vi "单轴运动.vi"() -> ()   [LabVIEW 2012]
panel:
  in  "停止速度":dbl=100.0
  out "运行曲线图 2":cluster{dbl[], i32[]}[](graph)
  out "运行时间":dbl
  out "当前状态":string
  out "当前速度":dbl
  out "当前位置":i32
  out "运行曲线图":cluster{dbl[], dbl[]}[](graph)
  in  "在线变位":bool
  in  "变位的位置值":i32=21000
  in  "平滑时间ms":dbl
  in  "减速时间s":dbl=0.5
  in  "加速时间s":dbl=0.5
  in  "运行速度":dbl=100000.0
  in  "起始速度":dbl=500.0
  in  "变速的速度值":dbl=1500.0
  in  "运动模式":enum32{"相对", "绝对"}(radio)
  in  "运动距离":i32=300000
  in  "运动方式":enum32{"点位", "连续"}(radio)
  in  "运动方向":enum32{"正向", "反向"}(radio)
  in  "在线变速":bool
  in  "退出":bool
  in  "紧急停止":bool
  in  "减速停止":bool
  in  "运行":bool
  in  "轴号选择":T1(ring)
  in  "脉冲清零":bool
  in  "卡号选择":u16(ring) items=["0"]
  out "init":bool
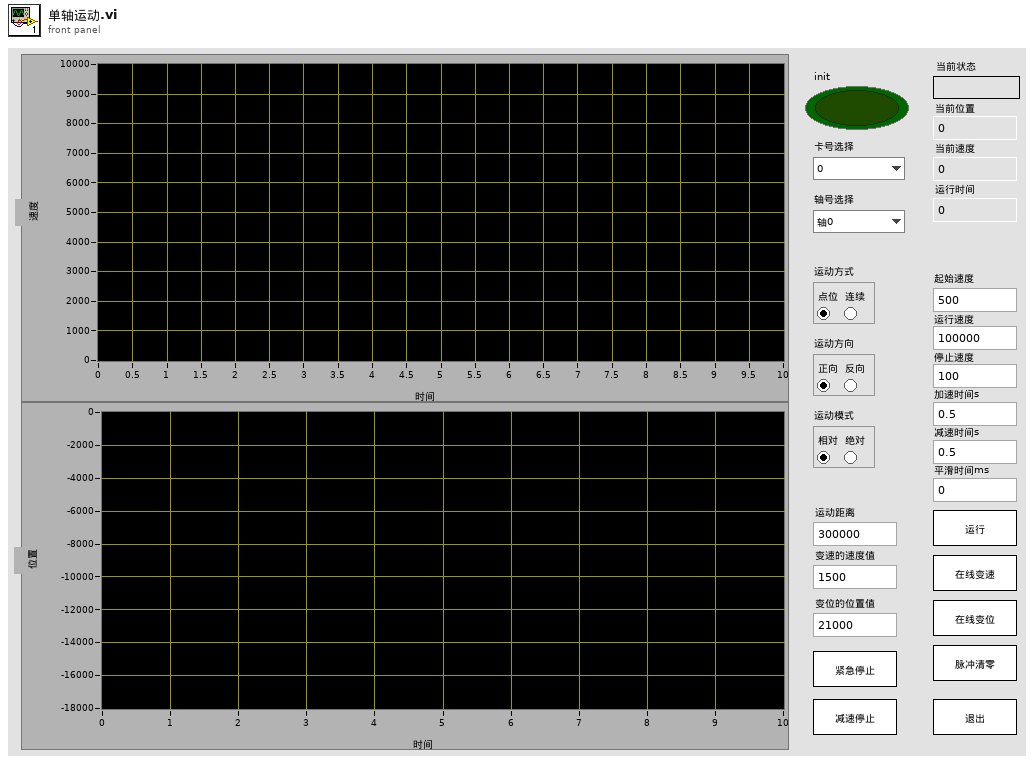
[diagram p1: front panel]
types:
  T1 = enum16{"轴0", "轴1", "轴2", "轴3", "轴4", "轴5", "轴6", "轴7"}
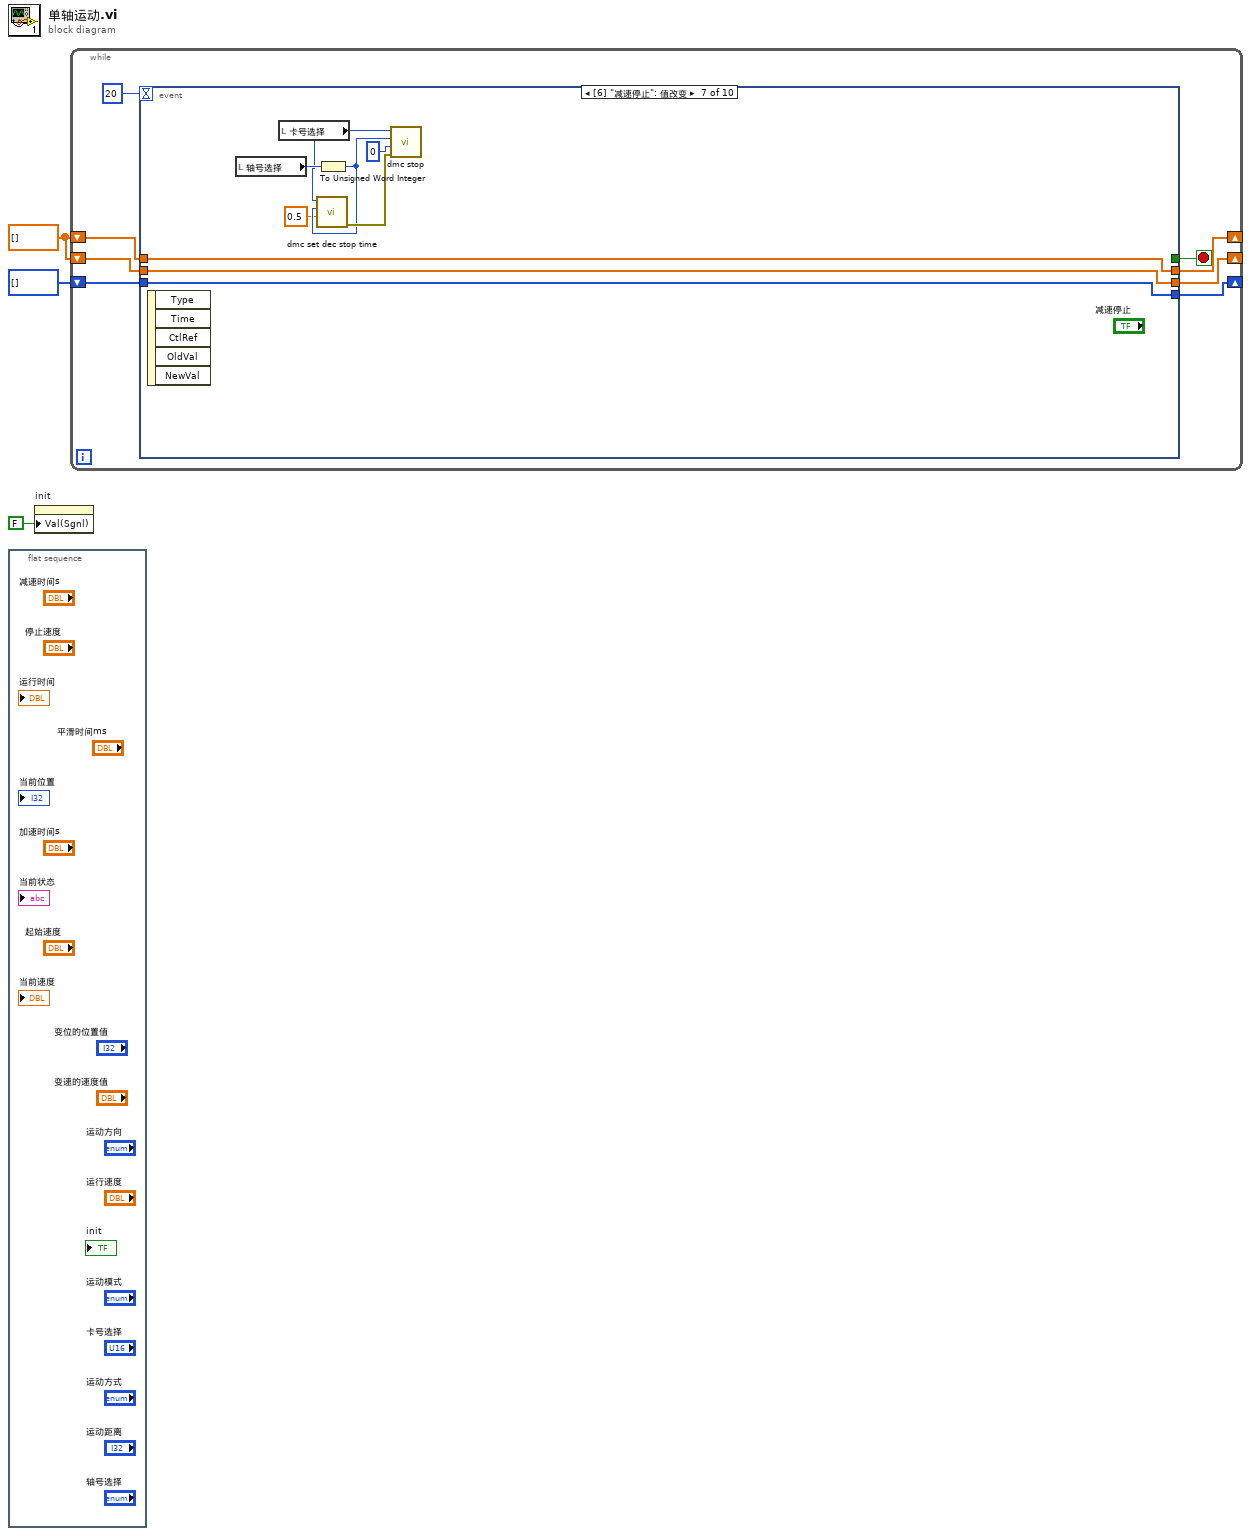
[diagram p0: block diagram]
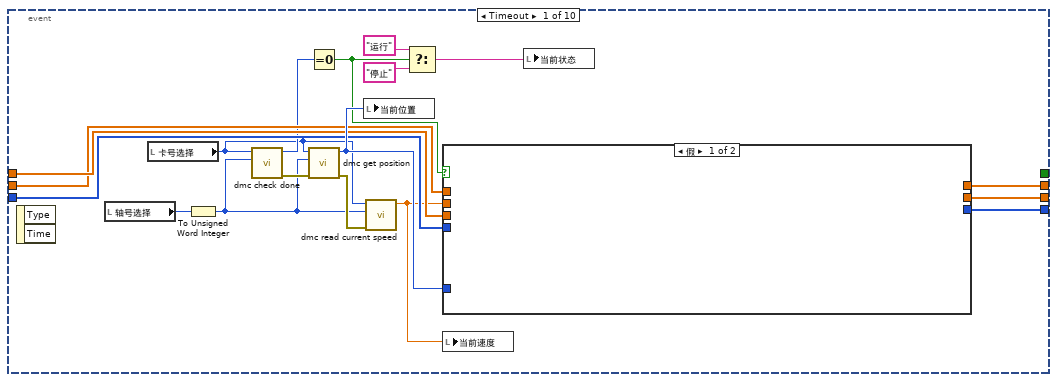
[diagram p2: hidden frame]
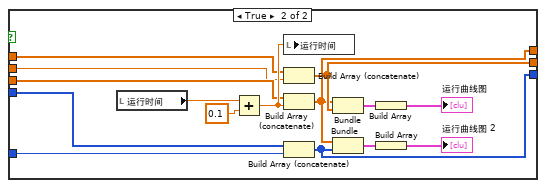
[diagram p3: hidden frame]
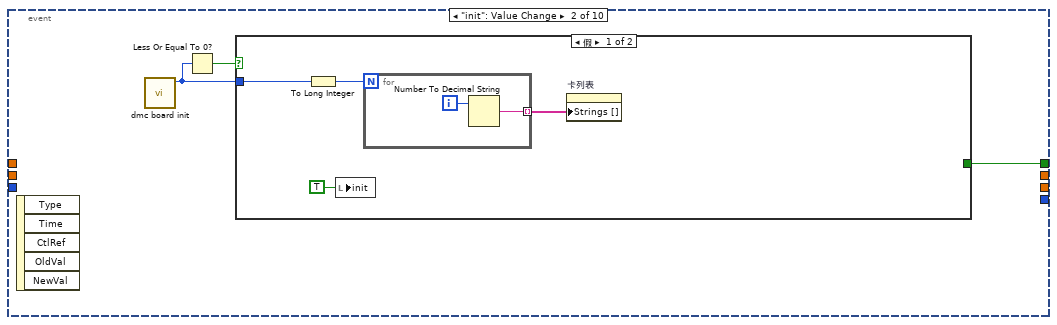
[diagram p4: hidden frame]
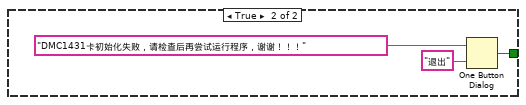
[diagram p5: hidden frame]
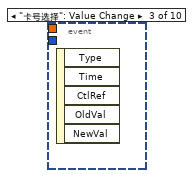
[diagram p6: hidden frame]
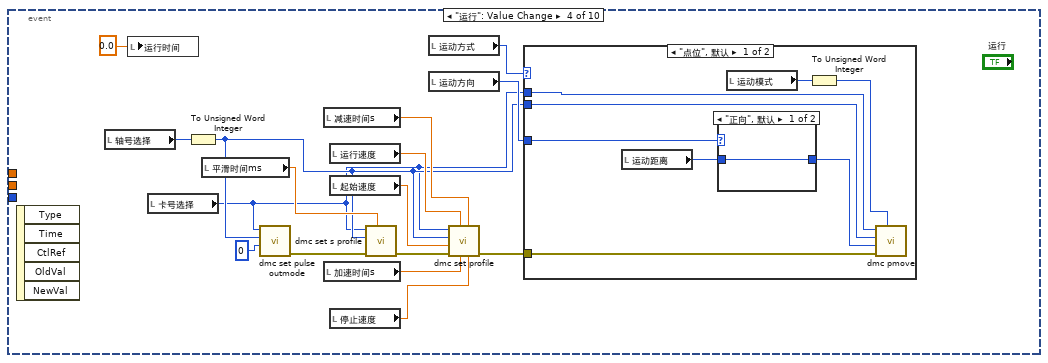
[diagram p7: hidden frame]
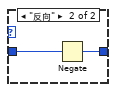
[diagram p8: hidden frame]
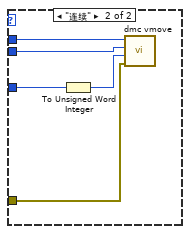
[diagram p9: hidden frame]
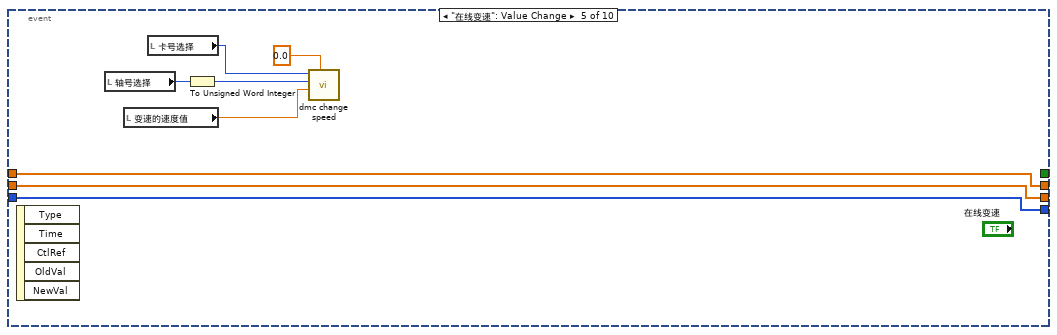
[diagram p10: hidden frame]
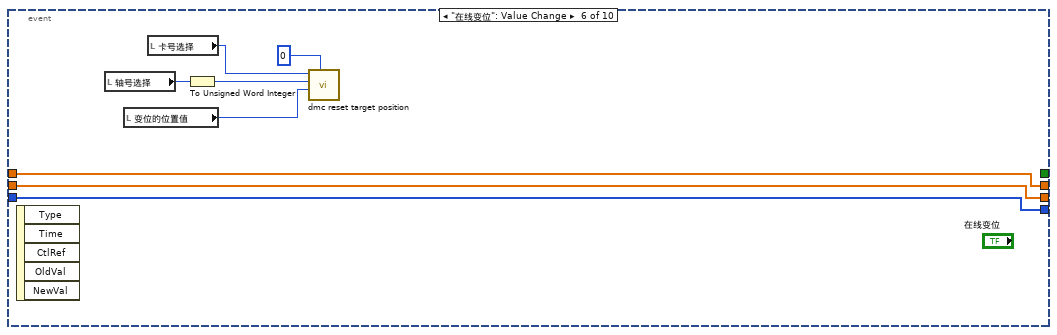
[diagram p11: hidden frame]
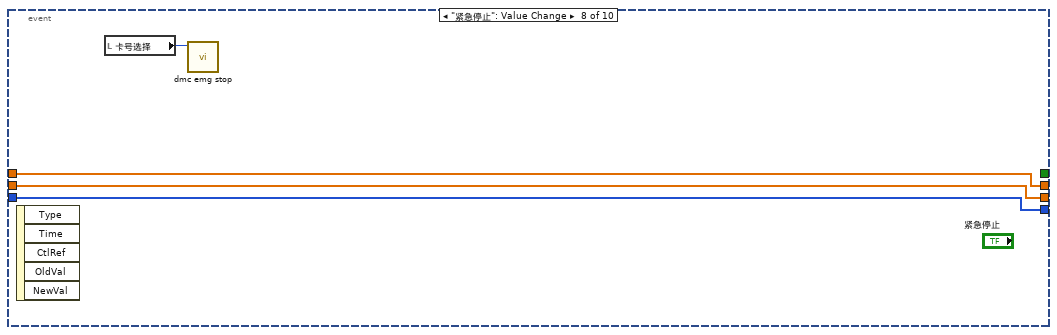
[diagram p12: hidden frame]
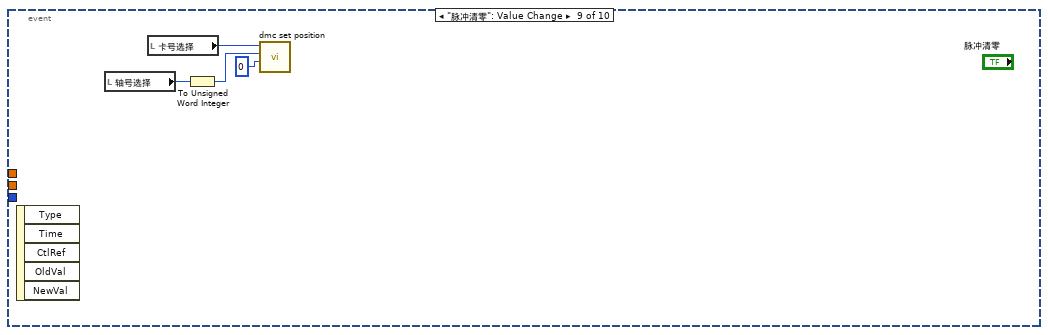
[diagram p13: hidden frame]
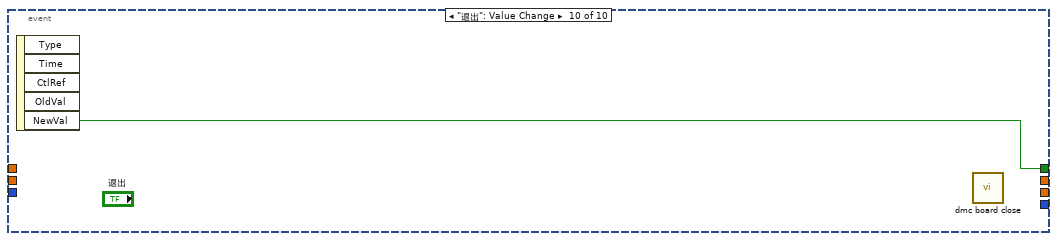
[diagram p14: hidden frame]
diagram:
  w1 = dbl[] []
  n1 = flat-sequence {
    frame #0 {
    }
  }
  n2 = property on="init" class="Bool (严格)"("Val(Sgnl)"=FALSE ("值(信号)")) -> ()  [unwired: 2 in, 2 out]
  n3 = while {
    shift-right: [w9] -> _
    shift-left: w1 -> [w8]
    shift-right: [w7] -> _
    shift-left: i32[] [] -> [w6]
    shift-right: [w4] -> _
    shift-left: w1 -> [w5]
    stop <- w11 stop-if-true
    n4 = event shown="[6] \"减速停止\": 值改变" {
      selector: _ -> [_ _ _ _ _ _ _ _ _ _]
      dyn-events: _ -> [_ _ _ _ _ _ _ _ _ _]
      timeout: 20 -> [_ _ _ _ _ _ _ _ _ _]
      tunnel: [_ w46 _ _ _ _ _ _ _ w122] -> w11
      tunnel: [w24 _ _ _ w95 w103 w112 w117 _ _] -> w9
      tunnel: w8 -> [w23 _ _ _ w95 w103 w112 w117 _ _]
      tunnel: [w22 _ _ _ w94 w102 w111 w116 _ _] -> w7
      tunnel: w6 -> [w21 _ _ _ w94 w102 w111 w116 _ _]
      tunnel: w5 -> [w20 _ _ _ w93 w101 w110 w115 _ _]
      tunnel: [w19 _ _ _ w93 w101 w110 w115 _ _] -> w4
      event Timeout {
        n5 = event-data() -> ()  [unwired: 1 in, 2 out]
        n6 = local read "轴号选择"() -> (w29:T1)
        n7 = local read "卡号选择"() -> (w13:u16)
        n8 = To Unsigned Word Integer(number=w29) -> (unsigned 16bit integer=w12:u16)
        n9 = call "dmc check done.vi"("axis"=w12, "CardNo"=w13) -> ("error out"=w15:errorcluster, "function return"=w16:i16)  [unwired: 8 in]
        n10 = Equal To 0?(x=w16) -> (x = 0?=w17:bool)
        n11 = call "dmc get position.vi"("error in (no error)"=w15, "axis"=w12, "CardNo"=w13) -> ("error out"=w14:errorcluster, "function return"=w25:i32)  [unwired: 7 in]
        n12 = local write "当前位置"(w25) -> ()
        n13 = call "dmc read current speed.vi"("error in (no error)"=w14, "axis"=w12, "CardNo"=w13) -> ("function return"=w18:dbl)  [unwired: 7 in, 1 out]
        n14 = Select(t="运行" ("当前状态"), s=w17, f="停止" ("当前状态")) -> (s? t:f=w28:string)
        n15 = case shown="假" w17 {
          tunnel: w25 -> [_ w40]
          tunnel: [_ w34] -> w24
          tunnel: w23 -> [_ w41]
          tunnel: [_ w38] -> w22
          tunnel: w21 -> [_ w39]
          tunnel: w20 -> [_ w37]
          tunnel: [_ w35] -> w19
          tunnel: w18 -> [_ w36]
          frame False {
          }
          frame True {
            n16 = local read "运行时间"() -> (w44:dbl)
            n17 = Add(x=w44, y=0.1) -> (x+y=w42:dbl)
            n18 = local write "运行时间"(w42) -> ()
            n19 = Build Array (concatenate)(w37, w36) -> (w35:dbl[])
            n20 = Build Array (concatenate)(w41, w42) -> (w34:dbl[])
            n21 = Build Array (concatenate)(w39, w40) -> (w38:i32[])
            n22 = Bundle(w34, w35) -> (w33:cluster{dbl[], dbl[]})  [unwired: 1 in]
            n23 = Bundle(w34, w38) -> (w30:cluster{dbl[], i32[]})  [unwired: 1 in]
            n24 = Build Array(w33) -> (→"运行曲线图":cluster{dbl[], dbl[]}[])
            n25 = Build Array(w30) -> (→"运行曲线图 2":cluster{dbl[], i32[]}[])
          }
        }
        n26 = local write "当前速度"(w18) -> ()
        n27 = local write "当前状态"(w28) -> ()
      }
      event "init": Value Change {
        n28 = event-data() -> ()  [unwired: 1 in, 5 out]
        n29 = call "dmc board init.vi"() -> ("function return"=w45:i16)  [unwired: 10 in, 1 out]
        n30 = Less Or Equal To 0?(x=w45) -> (x <= 0?=w47:bool)
        n31 = case shown="假" w47 {
          tunnel: [_ w54] -> w46
          tunnel: w45 -> [w51 _]
          frame False {
            n32 = To Long Integer(number=w51) -> (32bit integer=w50:i32)
            n33 = local write "init"(TRUE ("init")) -> ()
            n34 = for {
              N: w50 -> [_]
              tunnel: [w52] -> w49 mode=indexing
              i -> [w53]
              n35 = Number To Decimal String(number=w53) -> (decimal integer string=w52:string)  [unwired: 1 in]
            }
            n36 = property on="卡列表" class="Ring (严格)"("Strings []"=w49) -> ()  [unwired: 2 in, 2 out]
          }
          frame True {
            n37 = One Button Dialog(message="DMC1431卡初始化失败，请检查后再尝试运行程序，谢谢！！！" ("消息"), button name ("OK")="退出" ("按钮名称（“确定”）")) -> (true=w54:bool)
          }
        }
      }
      event "卡号选择": Value Change {
        n38 = event-data() -> ()  [unwired: 1 in, 5 out]
      }
      event "运行": Value Change {
        n39 = event-data() -> ()  [unwired: 1 in, 5 out]
        n40 = local read "轴号选择"() -> (w72:T1)
        n41 = local write "运行时间"(0.0 ("运行时间")) -> ()
        n42 = local read "卡号选择"() -> (w57:u16)
        n43 = To Unsigned Word Integer(number=w72) -> (unsigned 16bit integer=w58:u16)
        n44 = local read "平滑时间ms"() -> (w59:dbl)
        n45 = call "dmc set pulse outmode.vi"("outmode"=u16 0, "axis"=w58, "CardNo"=w57) -> ("error out"=w65:errorcluster)  [unwired: 7 in, 1 out]
        n46 = local read "减速时间s"() -> (w61:dbl)
        n47 = local read "加速时间s"() -> (w60:dbl)
        n48 = local read "运行速度"() -> (w62:dbl)
        n49 = local read "起始速度"() -> (w63:dbl)
        n50 = local read "停止速度"() -> (w68:dbl)
        n51 = call "dmc set s profile.vi"("s_para"=w59, "error in (no error)"=w65, "axis"=w58, "CardNo"=w57) -> ("error out"=w64:errorcluster)  [unwired: 6 in, 1 out]
        n52 = local read "运动方式"() -> (w71:enum32{"点位", "连续"})
        n53 = local read "运动方向"() -> (w70:enum32{"正向", "反向"})
        n54 = call "dmc set profile.vi"("stop_vel"=w68, "Tdec"=w61, "Tacc"=w60, "Max_Vel"=w62, "error in (no error)"=w64, "Min_Vel"=w63, "axis"=w58, "CardNo"=w57) -> ("error out"=w67:errorcluster)  [unwired: 2 in, 1 out]
        n55 = case shown="\"点位\", 默认" w71 {
          tunnel: w70 -> [w79 w88]
          tunnel: w67 -> [w73 w85]
          tunnel: w58 -> [w77 w84]
          tunnel: w57 -> [w76 w87]
          frame "点位", Default {
            n56 = local read "运动距离"() -> (w78:i32)
            n57 = case shown="\"正向\", 默认" w79 {
              tunnel: w78 -> [w81 w83]
              tunnel: [w81 w82] -> w75
              frame "正向", Default {
              }
              frame "反向" {
                n58 = Negate(x=w83) -> (-x=w82:i32)
              }
            }
            n59 = local read "运动模式"() -> (w80:enum32{"相对", "绝对"})
            n60 = To Unsigned Word Integer(number=w80) -> (unsigned 16bit integer=w74:u16)
            n61 = call "dmc pmove.vi"("posi_mode"=w74, "error in (no error)"=w73, "dist"=w75, "axis"=w77, "CardNo"=w76) -> ()  [unwired: 5 in, 2 out]
          }
          frame "连续" {
            n62 = To Unsigned Word Integer(number=w88) -> (unsigned 16bit integer=w86:u16)
            n63 = call "dmc vmove.vi"("error in (no error)"=w85, "dir"=w86, "axis"=w84, "CardNo"=w87) -> ()  [unwired: 6 in, 2 out]
          }
        }
      }
      event "在线变速": Value Change {
        n64 = event-data() -> ()  [unwired: 1 in, 5 out]
        n65 = local read "轴号选择"() -> (w96:T1)
        n66 = local read "变速的速度值"() -> (w90:dbl)
        n67 = local read "卡号选择"() -> (w91:u16)
        n68 = To Unsigned Word Integer(number=w96) -> (unsigned 16bit integer=w92:u16)
        n69 = call "dmc change speed.vi"("Taccdec"=0.0, "Curr_Vel"=w90, "axis"=w92, "CardNo"=w91) -> ()  [unwired: 6 in, 2 out]
      }
      event "在线变位": Value Change {
        n70 = event-data() -> ()  [unwired: 1 in, 5 out]
        n71 = local read "轴号选择"() -> (w104:T1)
        n72 = local read "变位的位置值"() -> (w98:i32)
        n73 = local read "卡号选择"() -> (w100:u16)
        n74 = To Unsigned Word Integer(number=w104) -> (unsigned 16bit integer=w99:u16)
        n75 = call "dmc reset target position.vi"("posi_mode"=u16 0, "dist"=w98, "axis"=w99, "CardNo"=w100) -> ()  [unwired: 6 in, 2 out]
      }
      event "减速停止": Value Change {
        n76 = event-data() -> ()  [unwired: 1 in, 5 out]
        n77 = local read "轴号选择"() -> (w113:T1)
        n78 = local read "卡号选择"() -> (w107:u16)
        n79 = To Unsigned Word Integer(number=w113) -> (unsigned 16bit integer=w106:u16)
        n80 = call "dmc set dec stop time.vi"("stop_time"=0.5, "axis"=w106, "CardNo"=w107) -> ("error out"=w108:errorcluster)  [unwired: 7 in, 1 out]
        n81 = call "dmc stop.vi"("error in (no error)"=w108, "stop_mode"=u16 0, "axis"=w106, "CardNo"=w107) -> ()  [unwired: 6 in, 2 out]
      }
      event "紧急停止": Value Change {
        n82 = event-data() -> ()  [unwired: 1 in, 5 out]
        n83 = local read "卡号选择"() -> (w114:u16)
        n84 = call "dmc emg stop.vi"("CardNo"=w114) -> ()  [unwired: 9 in, 2 out]
      }
      event "脉冲清零": Value Change {
        n85 = event-data() -> ()  [unwired: 1 in, 5 out]
        n86 = local read "轴号选择"() -> (w121:T1)
        n87 = local read "卡号选择"() -> (w120:u16)
        n88 = To Unsigned Word Integer(number=w121) -> (unsigned 16bit integer=w119:u16)
        n89 = call "dmc set position.vi"("current_position"=0, "axis"=w119, "CardNo"=w120) -> ()  [unwired: 7 in, 2 out]
      }
      event "退出": Value Change {
        n90 = event-data() -> ("NewVal"=w122:bool)  [unwired: 1 in, 4 out]
        n91 = call "dmc board close.vi"() -> ()  [unwired: 10 in, 2 out]
      }
    }
  }
